vi "fsk_test3.vi"(0 "total bits (128)":i32=128, 1 "symbol rate (Hz)":dbl=1.0 format="%.2f", 2 "samples per symbol (16)":i32=16, 3 "carrier frequency (Hz)":dbl min=-0.5 max=0.5 format="%.2f", 4 "FSK deviation (Hz)":dbl=150000.0 format="%.2p", 5 "pulse shaping filter (none)":T3(ring), 6 "Sync Words":i32[](array[numeric]), 7 "filter parameter":dbl=0.5 format="%.2f", 8 "Preamble Length":u32, 9 "filter length (symbols)":i32=8, 10 "symbol phase continuity":enum16{"continuous", "discontinuous"}(ring), 11 "reset? (T)":bool=TRUE) -> (13 "output bit stream":i8[](array[numeric]) caption="key bit sequence", 14 "upconverted waveform (complex)":T2 {"Y" format="%.3f"; "dt" format="%^.2e"; "t0" format="%.4f"}, 15 "FSK system parameters":T1 {"symbol map" format="%.2f"}, 16 "output cluster":T2={"t0"=0.0, "dt"=1.0, "Y"=[]} {"Y" format="%.3f"; "dt" format="%^.2e"; "t0" format="%.4f"}, 17 "pulse shaping filter coefficients":dbl[](array[numeric]) format="%.2f", 18 "matched filter coefficients":dbl[](array[numeric]) format="%.2f", 19 "error out":errorcluster)   [LabVIEW 2012]
uses:
  <vilib>/addons/Modulation/Analog/controls/Complex Data Waveform.ctl
  <vilib>/addons/Modulation/Digital/General/MT Generate FSK System Parameters(M).vi
  <vilib>/addons/Modulation/Analog/MT Upconvert Baseband (Complex).vi
  <vilib>/addons/Modulation/niDMT.lvlib
  <vilib>/addons/Modulation/niAMT.lvlib
panel:
  out "message":string=" INSTRUCTIONS:\r\rNormal Use:  When using subVIs that incorporate the error in/error out (or error I/O) structure, place this handler where you want to inform the user of an error, typically at the end of the I/O data path, as the last action of the program.  If the error in error? is ERROR, the handler creates a message describing the error and its source.  If the type of dialog = 1 (default), the message is displayed to the user, who can only acknowedge it.  If the type = 2, the user can acknowledge the message or abort execution; aborting a program with active I/O is not recommended.  If the type = 0, no message is displayed; this is used to process the error programmatically, and the error out cluster elements are wired to individual terminals for that reason.  \r\rOther Use:\n\r\nlocal testing.  To test the error code of a subVI or function that does not have the error I/O structure, you can wire its error code and a source string to the local error code and error source inputs.  If error in error? indicates no error and error code is not equal to 0, the local code and source are substituted for the error in values, and error? is set TRUE (ERROR)."
  out "FFT - (RMS)":dbl[](graph)
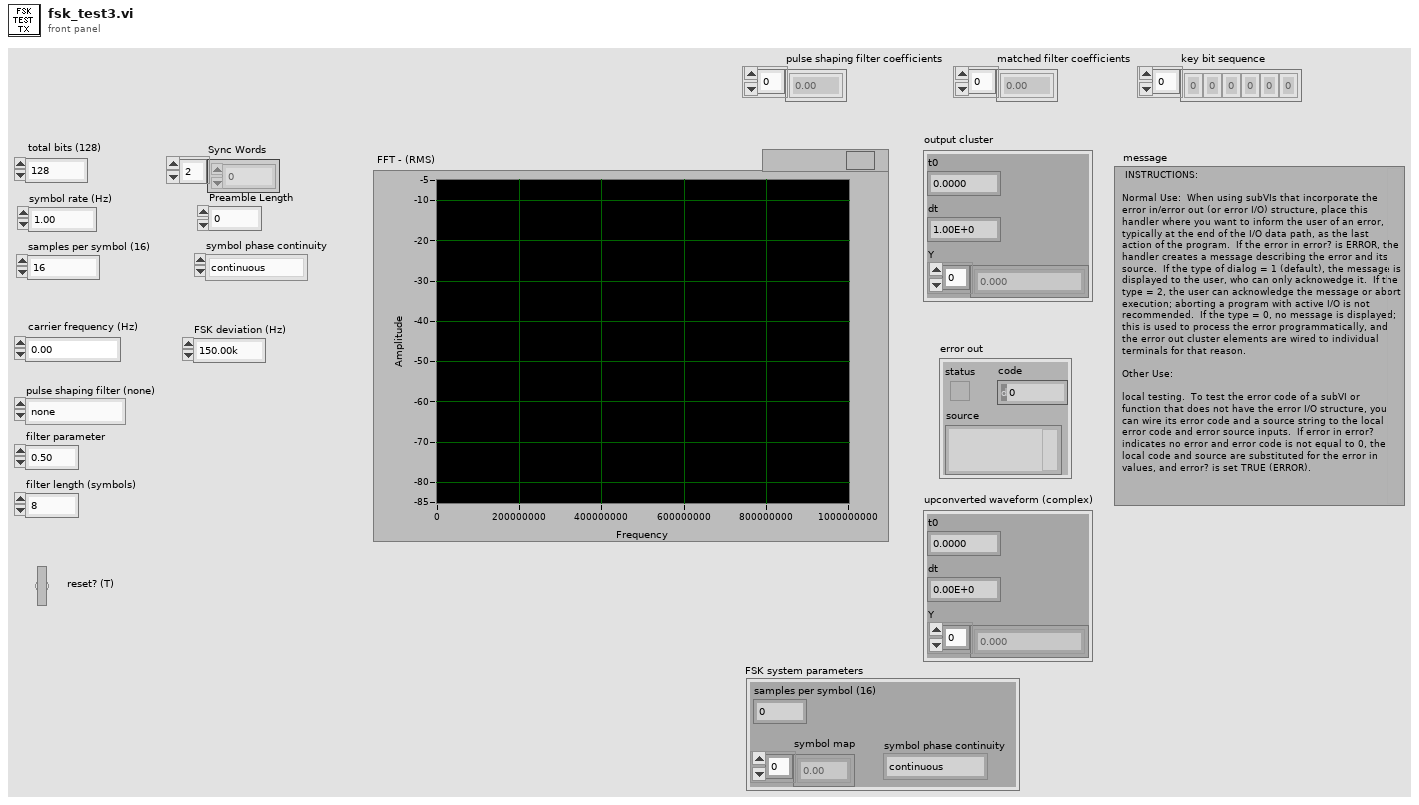
[diagram p1: front panel]
types:
  T1 = cluster{"samples per symbol (16)":i32, "symbol map":dbl[], "symbol phase continuity":enum16{"continuous", "discontinuous"}}
  T2 = typedef "niAMT.lvlib/Complex Data Waveform.ctl" = cluster{"t0":dbl, "dt":dbl, "Y":cdb[]}
  T3 = enum16{"none", "Raised Cosine", "Root Raised Cos", "Gaussian"}
  T4 = enum16{"FSK", "PSK", "QAM", "MSK", "PAM", "ASK", "CPM"}
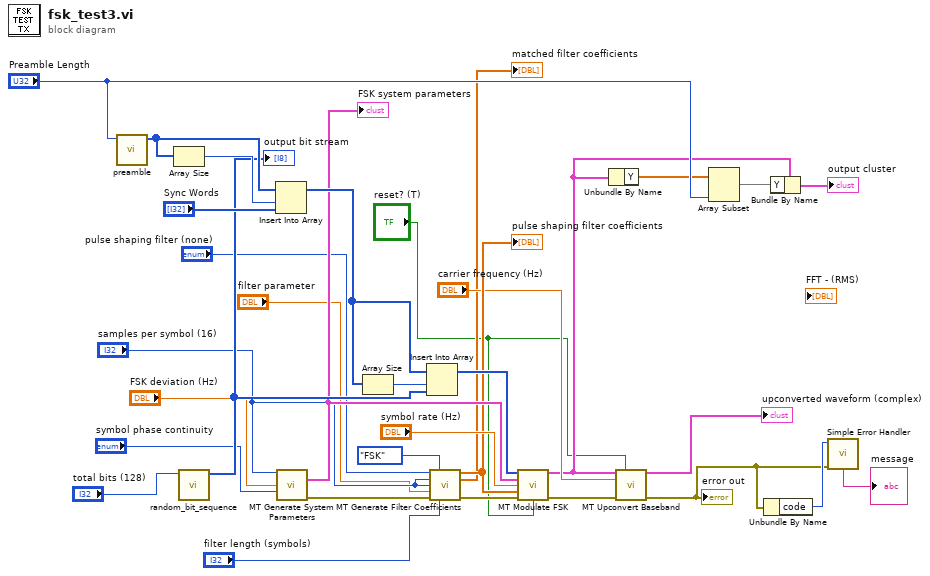
[diagram p0: block diagram]
diagram:
  n1 = call "preamble.vi"("Preamble Length (bits)"="Preamble Length") -> ("Preamble"=w31:i32[])  [unwired: 10 in]
  n2 = Array Size(array=w31) -> (size(s)=w30:i32)
  n3 = call "random_bit_sequence.vi"("Length"="total bits (128)") -> ("Bit Sequence"=w27:i8[])  [unwired: 10 in]
  "output bit stream" <- w27
  n4 = Insert Into Array(array=w31, index=w30, new element="Sync Words") -> (w29:i32[])
  n5 = call-poly <vilib>:"MT Generate System Parameters.vi"("samples per symbol (16)"="samples per symbol (16)", "FSK deviation (Hz)"="FSK deviation (Hz)", "symbol phase continuity"="symbol phase continuity") -> ("FSK system parameters"=w23:T1, "error out"=w19:errorcluster)  [unwired: 10 in, 1 out]
  "FSK system parameters" <- w23
  n6 = Array Size(array=w29) -> (size(s)=w28:i32)
  n7 = Insert Into Array(array=w29, index=w28, new element=w27) -> (w26:i32[])
  n8 = call <vilib>:"MT Generate Filter Coefficients.vi"("pulse shaping filter (none)"="pulse shaping filter (none)", "modulation type"=T4."FSK", "pulse shaping samples per symbol (16)"="samples per symbol (16)", "matched samples per symbol (16)"="samples per symbol (16)", "filter parameter"="filter parameter", "error in (no error)"=w19, "filter length (symbols)"="filter length (symbols)") -> ("pulse shaping filter coefficients"=w17:dbl[], "matched filter coefficients"=→"matched filter coefficients":dbl[], "error out"=w18:errorcluster)  [unwired: 6 in]
  "pulse shaping filter coefficients" <- w17
  n9 = call <vilib>:"MT Modulate FSK.vi"("input bit stream"=w26, "FSK system parameters"=w23, "symbol rate (Hz)"="symbol rate (Hz)", "pulse shaping filter coefficients"=w17, "error in (no error)"=w18, "reset? (T)"="reset? (T)") -> ("output complex waveform"=w5:T2, "error out"=w13:errorcluster)  [unwired: 7 in, 1 out]
  n10 = Unbundle By Name(w5) -> ("Y"=w2:cdb[])
  n11 = call-poly <vilib>:"MT Upconvert Baseband.vi"("complex waveform"=w5, "reset? (F)"="reset? (T)", "carrier frequency (Hz)"="carrier frequency (Hz)", "error in (no error)"=w13) -> ("upconverted waveform (complex)"=→"upconverted waveform (complex)":T2, "error out"=w4:errorcluster)  [unwired: 10 in]
  "error out" <- w4
  n12 = Array Subset(array=w2, length="Preamble Length") -> (w7:cdb[])  [unwired: 1 in]
  n13 = Unbundle By Name(w4) -> ("code"=w10:i32)
  n14 = Bundle By Name(cluster=w5, "Y"=w7) -> (→"output cluster":T2)
  n15 = call <vilib>:"Simple Error Handler.vi"("error code (no error:0)"=w10, "error in (no error)"=w4) -> ("message"=→"message":string)  [unwired: 3 in, 4 out]
